vi "ui_DataLog Query Tags.vi"(0 "prompt":string, 7 "database":string, 11 "value type (any)":enum16{"any", "number", "string"}(ring)) -> (4 "OK?":bool, 8 "tag":string[](array[string]))   [LabVIEW 2012]
doc: "Shows a convenient dialog for selecting a tag."
uses:
  typedefs/t_DataLog Tag Info List Methods.ctl
  served/DataLog Database Infos_srv.ctl
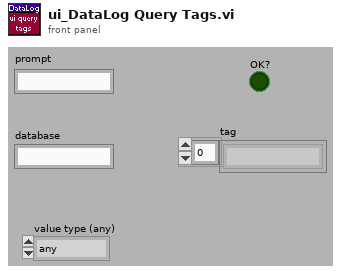
[diagram p1: front panel]
types:
  T1 = typedef "DataLog Database Infos_srv.ctl" = refnum<vi>
  T2 = typedef "t_DataLog Tag Info List Methods.ctl" = enum16{"initialize", "create", "create empty", "rename", "delete", "test tag", "get", "get by name", "get default", "get list", "get path", "get subsets", "set subsets", "set config", "set capacity", "#tags", "go live", "set unlocked", "set mirrored"}
  T3 = typedef "t_DataLog Tag Config.ctl" = cluster{"name":string, "unit":string, "temporal":T4, "value":T5, "index":i32, "capacity":i32, "is meta?":bool, "mincapacity":i32, "deadband":dbl, "limit delay":dbl, "format":T6, "precision":u8, "undefine":bool, "update":bool, "update period":u16, "expression":string, "description":string, "logging algorithm":T7, "logging parameters":dbl[]}
  T4 = typedef "t_DataLog Temporal Types.ctl" = enum16{"set&hold", "sample", "event"}
  T5 = typedef "t_DataLog Value Types.ctl" = enum16{"number", "string"}
  T6 = typedef "t_DataLog Numerical Format.ctl" = enum8{"fractional", "exponential", "engineering"}
  T7 = typedef "t_DataLog Logging Algorithms.ctl" = enum16{"nothing", "changes", "everything", "every Nth", "time threshold", "value threshold + prior", "t or v threshold", "t or v threshold + prior"}
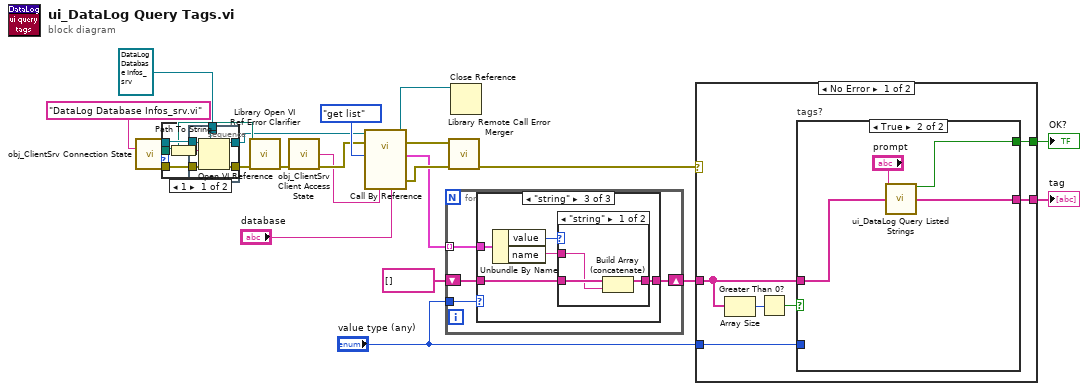
[diagram p0: block diagram]
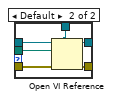
[diagram p2: hidden frame]
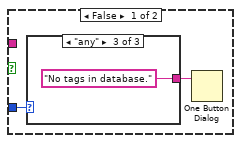
[diagram p3: hidden frame]
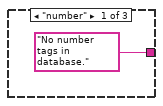
[diagram p4: hidden frame]
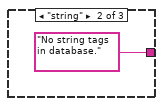
[diagram p5: hidden frame]
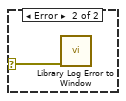
[diagram p6: hidden frame]
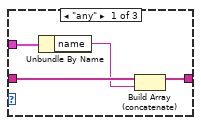
[diagram p7: hidden frame]
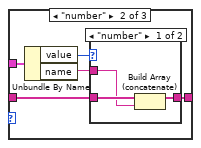
[diagram p8: hidden frame]
diagram:
  n1 = call "obj_ClientSrv Connection State.vi"("machine{connect}/VI{get state} name (local/no path resolution)"="DataLog Database Infos_srv.vi") -> ("server app ref"=w4:refnum<vi>, "resolved server path"=w3:path, "error out"=w2:errorcluster)  [unwired: 7 in, 5 out]
  n2 = stacked-sequence {
    tunnel: [w28] -> w1
    tunnel: [w27] -> w6
    tunnel: w2 -> [w26]
    tunnel: w4 -> [w25]
    tunnel: w3 -> [w24]
    tunnel: T1 refnum ("database infos") -> [w23]
    frame #0 {
      # "avoid LV8 complaints"
      n3 = Path to Array of Strings(0:w24) -> (2:w29:string[])  [unwired: 1 out]
      n4 = Array Size(array=w29) -> (size(s)=w30:i32)
      n5 = case shown="1" w30 {
        tunnel: w24 -> [w37 w43]
        tunnel: w25 -> [w35 w42]
        tunnel: [w33 w38] -> w28
        tunnel: [w31 w41] -> w27
        tunnel: w23 -> [w32 w40]
        tunnel: w26 -> [w34 w39]
        frame 1 {
          n6 = Path To String(path=w37) -> (string=w36:string)
          n7 = Open VI Reference(type specifier VI Refnum (for type only)=w32, application reference (local)=w35, vi path=w36, error in (no error)=w34) -> (vi reference=w33:T1, error out=w31:errorcluster)  [unwired: 2 in]
        }
        frame Default {
          n8 = Open VI Reference(type specifier VI Refnum (for type only)=w40, application reference (local)=w42, vi path=w43, error in (no error)=w39) -> (vi reference=w38:T1, error out=w41:errorcluster)  [unwired: 2 in]
        }
      }
    }
  }
  n9 = call "Library Open VI Ref Error Clarifier.vi"("VI path"=w3, "called VI error (no error)"=w6) -> ("error out"=w17:errorcluster)  [unwired: 13 in]
  n10 = call "obj_ClientSrv Client Access State.vi"("error in (no error)"=w17) -> ("certificate"=w12:string, "error out"=w21:errorcluster)  [unwired: 13 in]
  n11 = call-by-ref "?"(reference=w1, error in=w21, "method"=t_DataLog_Tag_Info_List_Methods."get list", "certificate in"=w12, "database (current)"="database") -> (reference out=w14:T1, error out=w19:errorcluster, "tag config list"=w18:T3[], 15:"error out"=w20:errorcluster)  [unwired: 7 in, 4 out]
  n12 = for {
    tunnel: w18 -> [w47] mode=indexing
    tunnel: "value type (any)" -> [w46]
    shift-right: [w44] -> w9
    shift-left: string[] [] -> [w45]
    n13 = case shown="\"string\"" w46 {
      tunnel: w47 -> [w51 w56 w65]
      tunnel: w45 -> [w50 w54 w63]
      tunnel: [w48 w53 w62] -> w44
      frame "any" {
        n14 = Unbundle By Name(w51) -> ("name"=w49:string)
        n15 = Build Array (concatenate)(w50, w49) -> (w48:string[])
      }
      frame "number" {
        n16 = Unbundle By Name(w56) -> ("value"=w55:T5, "name"=w52:string)
        n17 = case shown="\"number\"" w55 {
          tunnel: w54 -> [w58 w60]
          tunnel: [w59 w60] -> w53
          tunnel: w52 -> [w57 _]
          frame "number" {
            n18 = Build Array (concatenate)(w58, w57) -> (w59:string[])
          }
          frame "string" {
          }
        }
      }
      frame "string" {
        n19 = Unbundle By Name(w65) -> ("value"=w64:T5, "name"=w61:string)
        n20 = case shown="\"string\"" w64 {
          tunnel: w63 -> [w67 w69]
          tunnel: [w68 w69] -> w62
          tunnel: w61 -> [w66 _]
          frame "string" {
            n21 = Build Array (concatenate)(w67, w66) -> (w68:string[])
          }
          frame "number" {
          }
        }
      }
    }
  }
  n22 = call "Library Remote Call Error Merger.vi"("call by reference node error"=w19, "called VI error (no error)"=w20) -> ("error out"=w7:errorcluster)  [unwired: 13 in]
  n23 = Close Reference(reference=w14) -> ()  [unwired: 1 in, 1 out]
  n24 = case shown="No Error" w7 {
    selector: w7 -> [_ w85]
    tunnel: [w75 _] -> w16
    tunnel: [w74 _] -> w15
    tunnel: w9 -> [w71 _]
    tunnel: "value type (any)" -> [w70 _]
    frame No Error {
      n25 = Array Size(array=w71) -> (size(s)=w73:i32)
      n26 = Greater Than 0?(x=w73) -> (x > 0?=w72:bool)
      n27 = case "tags?" shown="True" w72 {
        tunnel: [_ w84] -> w75
        tunnel: [_ w83] -> w74
        tunnel: w71 -> [_ w81]
        tunnel: w70 -> [w77 _]
        frame False {
          n28 = case shown="\"any\"" w77 {
            tunnel: ["No number tags in database." ("selected string") "No string tags in database." ("selected string") "No tags in database." ("selected string")] -> w76
            frame "number" {
            }
            frame "string" {
            }
            frame "any" {
            }
          }
          n29 = One Button Dialog(message=w76) -> ()  [unwired: 1 in, 1 out]
        }
        frame True {
          n30 = call "ui_DataLog Query Listed Strings.vi"("prompt"="prompt", "list of strings"=w81) -> ("OKed?"=w84:bool, "selected strings"=w83:string[])  [unwired: 12 in]
        }
      }
    }
    frame Error {
      n31 = call "Library Log Error to Window.vi"("error in (no error)"=w85) -> ()  [unwired: 13 in, 2 out]
    }
  }
  "tag" <- w15
  "OK?" <- w16
